vi "260520_demo_test_tryout_5spm.vi"() -> ()   [LabVIEW 2022 SP3]
uses:
  <vilib>/Analysis/baseanly.llb/Mean (DBL).vi
  <vilib>/express/express analysis/Spectral/Block/exnSpectralBlock spectral measurements peak poly.vi
  <vilib>/express/express analysis/Spectral/Block/exnSpectralBlock spectral measurements peak DDT.vi
  <vilib>/express/express analysis/Spectral/XNode/ExpressSpectralMeasurementsBlockNode.xnode
  <vilib>/Analysis/NI_AALBase.lvlib
panel:
  out "Waveform Graph":dynamicdata(graph)
  out "y":dbl
  out "mean 2":dbl format="%.8g"
  out "mean":dbl format="%.8g"
  out "Section 4":dynamicdata(graph) caption="Section"
  out "Section 3":dynamicdata(graph) caption="Section"
  out "Section 2":dynamicdata(graph) caption="Section"
  out "Section":dynamicdata(graph)
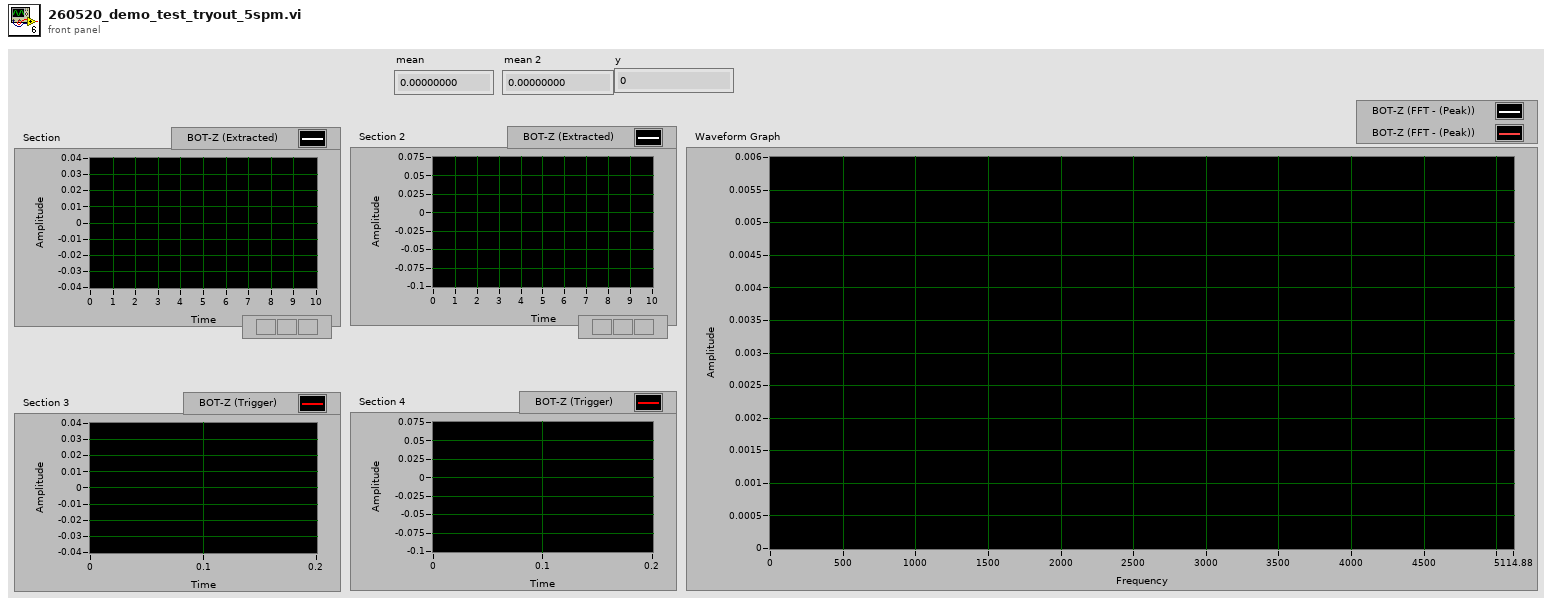
[diagram p1: front panel]
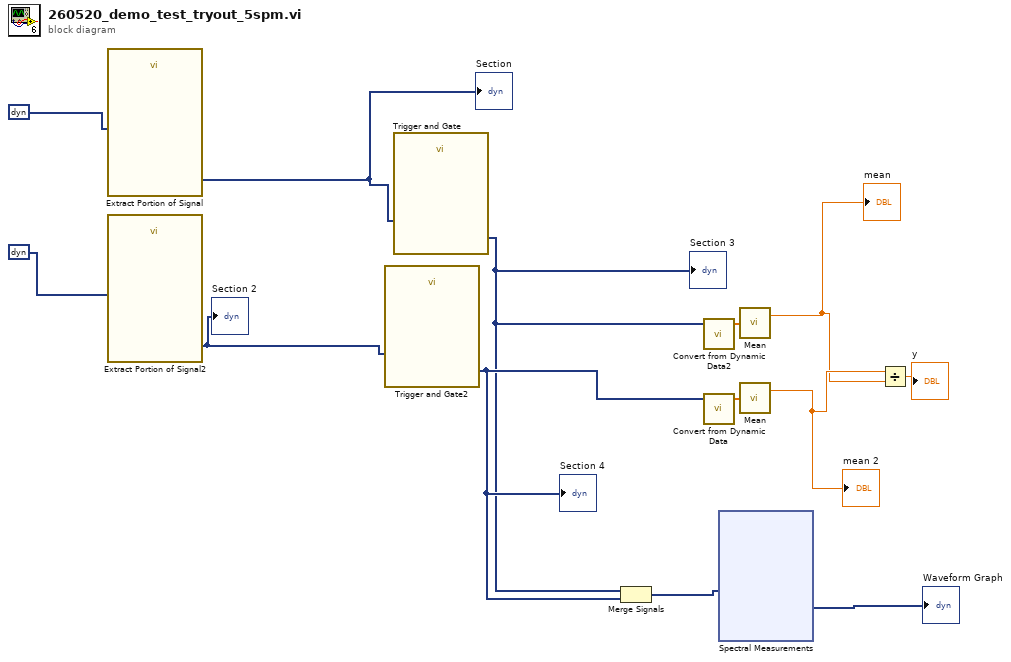
[diagram p0: block diagram]
diagram:
  n1 = call "Extract Portion of Signal"("Signals"=dynamicdata [{"t0"=timestamp(0 s since 1904-01-01), "dt"=9.765625e-05, "Y"=array[710000 elements], "attributes"=variant("NI_ChannelName"=variant(string "BOT-Z"), "NI_ExpIsRelativeTime"=variant(bool TRUE), "NI_ExpStartTimeStamp"=variant(timestamp timestamp(3862102967.667043 s since 1904-01-01)), "NI_ExpTimeStamp"=variant(timestamp timestamp(3862102967.667043 s since 1904-01-01)), "NI_ExpXDimension"=variant(string "t"), "NI_UnitDescription"=variant(string "g"))}] ("Waveform Graph 4")) -> ("Section"=w11:dynamicdata)  [unwired: 9 in, 1 out]
  "Section" <- w11
  n2 = call "Extract Portion of Signal2"("Signals"=dynamicdata [{"t0"=timestamp(0 s since 1904-01-01), "dt"=9.765625e-05, "Y"=array[270000 elements], "attributes"=variant("NI_ChannelName"=variant(string "BOT-Z"), "NI_ExpIsRelativeTime"=variant(bool TRUE), "NI_ExpStartTimeStamp"=variant(timestamp timestamp(3862102967.667043 s since 1904-01-01)), "NI_ExpTimeStamp"=variant(timestamp timestamp(3862103059.463918 s since 1904-01-01)), "NI_ExpXDimension"=variant(string "t"), "NI_UnitDescription"=variant(string "g"))}] ("Waveform Graph 3")) -> ("Section"=w10:dynamicdata)  [unwired: 9 in, 1 out]
  "Section 2" <- w10
  n3 = call "Trigger and Gate2"("Signals"=w10) -> ("Triggered Signals"=w5:dynamicdata)  [unwired: 7 in, 3 out]
  "Section 4" <- w5
  n4 = call "Trigger and Gate"("Signals"=w11) -> ("Triggered Signals"=w2:dynamicdata)  [unwired: 7 in, 3 out]
  "Section 3" <- w2
  n5 = Merge Signals(w2, w5) -> (w3:dynamicdata)
  n6 = call "Convert from Dynamic Data2"("Dynamic Data Type"=w2) -> ("Array"=w8:dbl[])  [unwired: 3 in]
  n7 = call "Convert from Dynamic Data"("Dynamic Data Type"=w5) -> ("Array"=w9:dbl[])  [unwired: 3 in]
  n8 = xnode "Spectral Measurements"("Signals"=w3) -> ("FFT - (Peak)"=→"Waveform Graph":dynamicdata)  [unwired: 1 in, 2 out]
  n9 = call-poly <vilib>:"Mean.vi"("X"=w8) -> ("mean"=w1:dbl)  [unwired: 1 out]
  "mean" <- w1
  n10 = call-poly <vilib>:"Mean.vi"("X"=w9) -> ("mean"=w7:dbl)  [unwired: 1 out]
  "mean 2" <- w7
  n11 = Divide(x=w7, y=w1) -> (x/y=→"y":dbl)
